vi "closeTDMS.vi"(8 "error in (no error)":errorcluster {"code" format="Error %.0f"}, 11 "filepath":refnum<k34>) -> (0 "error out":errorcluster {"code" format="Error %.0f"})   [LabVIEW 2017]
doc: "This VI closes and defrags a TDMS file."
uses:
  <vilib>/Utility/error.llb/Error Cluster From Error Code.vi
  <vilib>/ErrorRing/Error Ring.xnode
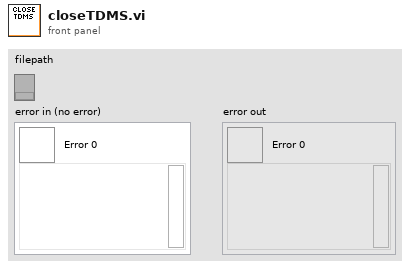
[diagram p1: front panel]
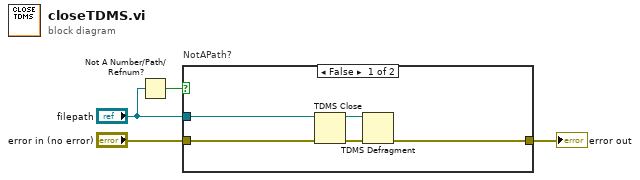
[diagram p0: block diagram]
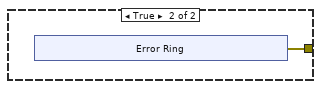
[diagram p2: hidden frame]
diagram:
  n1 = Not A Number/Path/Refnum?(number/path/refnum="filepath") -> (NaN/Path/Refnum?=w4:bool)
  n2 = case "NotAPath?" shown="False" w4 {
    tunnel: "error in (no error)" -> [w7 _]
    tunnel: [w6 w10] -> w2
    tunnel: "filepath" -> [w5 _]
    frame False {
      n3 = TDMS Close(8:w7, 11:w5) -> (0:w8:errorcluster, 3:w9:path)
      n4 = TDMS Defragment(4:w8, 7:w9) -> (0:w6:errorcluster)
    }
    frame True {
      n5 = xnode "Error Ring"() -> ("error out"=w10:errorcluster)
    }
  }
  "error out" <- w2
